vi "Set Physical Channel Property.vi"(0 "Session Handle in":T1, 5 "physical channels":refnum<k21>="$DefaultPhysChans", 7 "property":refnum<k21>, 9 "property value":bool, 11 "error in (no error)":errorcluster) -> (4 "Session Handle out":T1, 15 "error out":errorcluster)   [LabVIEW 2015]
uses:
  <vilib>/SLSC/SLSC.lvlib
  <vilib>/SLSC/Set Phys Chan Property (Bool).vi
  Relay Interface/RelayInterface.lvclass
  Relay Interface/Commit Buffer Action.ctl
  SLSC Session.lvclass
  Typedefs/Session Handle.ctl
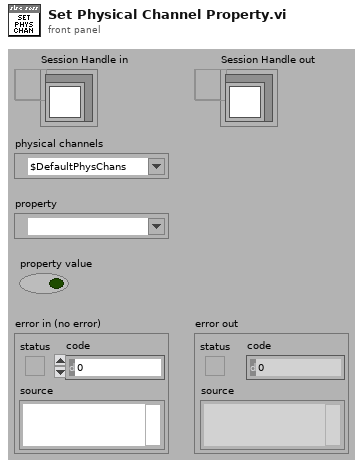
[diagram p1: front panel]
types:
  T1 = typedef "SLSC Switch.lvlib/SLSC Session.lvclass/Session Handle.ctl" = refnum<data-value>
  T2 = typedef "RelayInterface.lvclass/Commit Buffer Action.ctl" = enum16{"Get Session Buffer", "Add Transaction", "Clear Session Buffer", "Clear All"}
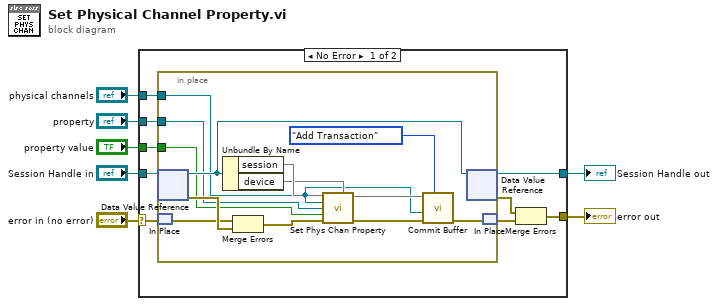
[diagram p0: block diagram]
diagram:
  n1 = case shown="No Error" "error in (no error)" {
    selector: "error in (no error)" -> [w11 w29]
    tunnel: "Session Handle in" -> [w16 w30]
    tunnel: [w15 w30] -> w6
    tunnel: [w12 w29] -> w5
    tunnel: "physical channels" -> [w10 _]
    tunnel: "property" -> [w9 _]
    tunnel: "property value" -> [w8 _]
    frame No Error {
      n2 = in-place {
        in-place-border: w10 -> [w19]
        in-place-border: w9 -> [w23]
        in-place-border: w8 -> [w22]
        n3 = in-place-dvr #1(w16) -> (w26:refnum<class "SLSC Session.lvclass">, w28:errorcluster)
        n4 = in-place-match #2(w11) -> (w27:errorcluster)
        n5 = Unbundle By Name(w26) -> ("session"=w25, "device"=w20)
        n6 = Merge Errors(w27, w28) -> (w24:errorcluster)
        n7 = call-poly <vilib>:"Set Phys Chan Property.vi"("session in"=w25, "physical channels"=w19, "property"=w23, "property value"=w22, "error in (no error)"=w24) -> ("error out"=w18:errorcluster)  [unwired: 9 in, 1 out]
        n8 = call "Commit Buffer.vi"("Action"=Commit_Buffer_Action."Add Transaction", "error in (no error)"=w18, "Transation String"=w19, "device name in"=w20) -> ("error out"=w17:errorcluster)  [unwired: 6 in, 1 out]
        n9 = in-place-dvr #1(w26) -> (w15:T1, w13:errorcluster)
        n10 = in-place-match #2(w17) -> (w14:errorcluster)
      }
      n11 = Merge Errors(w13, w14) -> (w12:errorcluster)
    }
    frame Error {
    }
  }
  "Session Handle out" <- w6
  "error out" <- w5
